vi "bigcryo-T-full.vi"() -> (2 "VTI [K]":dbl=1.4652, 3 "Spl [K]":dbl=1.6452)   [LabVIEW 2019]
uses:
  Global 2.vi
  <vilib>/Analysis/NI_AALPro.lvlib
panel:
  out "Stable?":bool
  out "read buffer":string
  in  "stop":bool
  out "Running Sequence":bool
  out "VTI Rate":dbl format="%#.3g"
  out "Rate":dbl format="%#.3g"
  in  "Rate":dbl
  in  "Reset Graph":bool
  in  "Ramp":bool
  in  "Go To":bool
  in  "Set Temp":dbl=1.6
  out "Range":dbl
  out "Spl":dbl(slide) scale=0.0..100.0
  out "VTI":dbl(slide) scale=0.0..100.0
  out "T":cluster{"X":dbl[], "Y":dbl[]}[](graph)=[{"X"=[158.55365709999998, 159.610163, 160.67648119999998, 161.7360579, 162.7961535, 163.85780699999998], "Y"=[1.4652, 1.4652, 1.4653, 1.4652, 1.4651, 1.4652]}, {"X"=[158.55365709999998, 159.610163, 160.67648119999998, 161.7360579, 162.7961535, 163.85780699999998], "Y"=[1.6459, 1.6456, 1.6455, 1.6454, 1.6452, 1.6452]}] caption="XY Graph"
  out "Set VTI [K]":dbl=1.2
  out "Set Spl [K]":dbl=1.6
  # "Heaters"
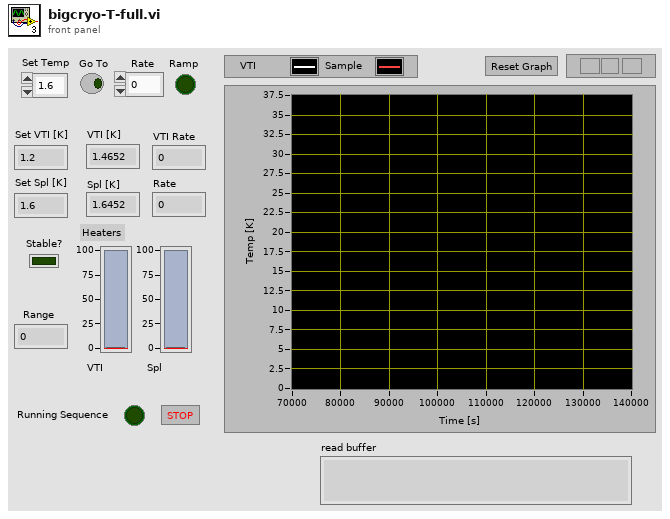
[diagram p1: front panel]
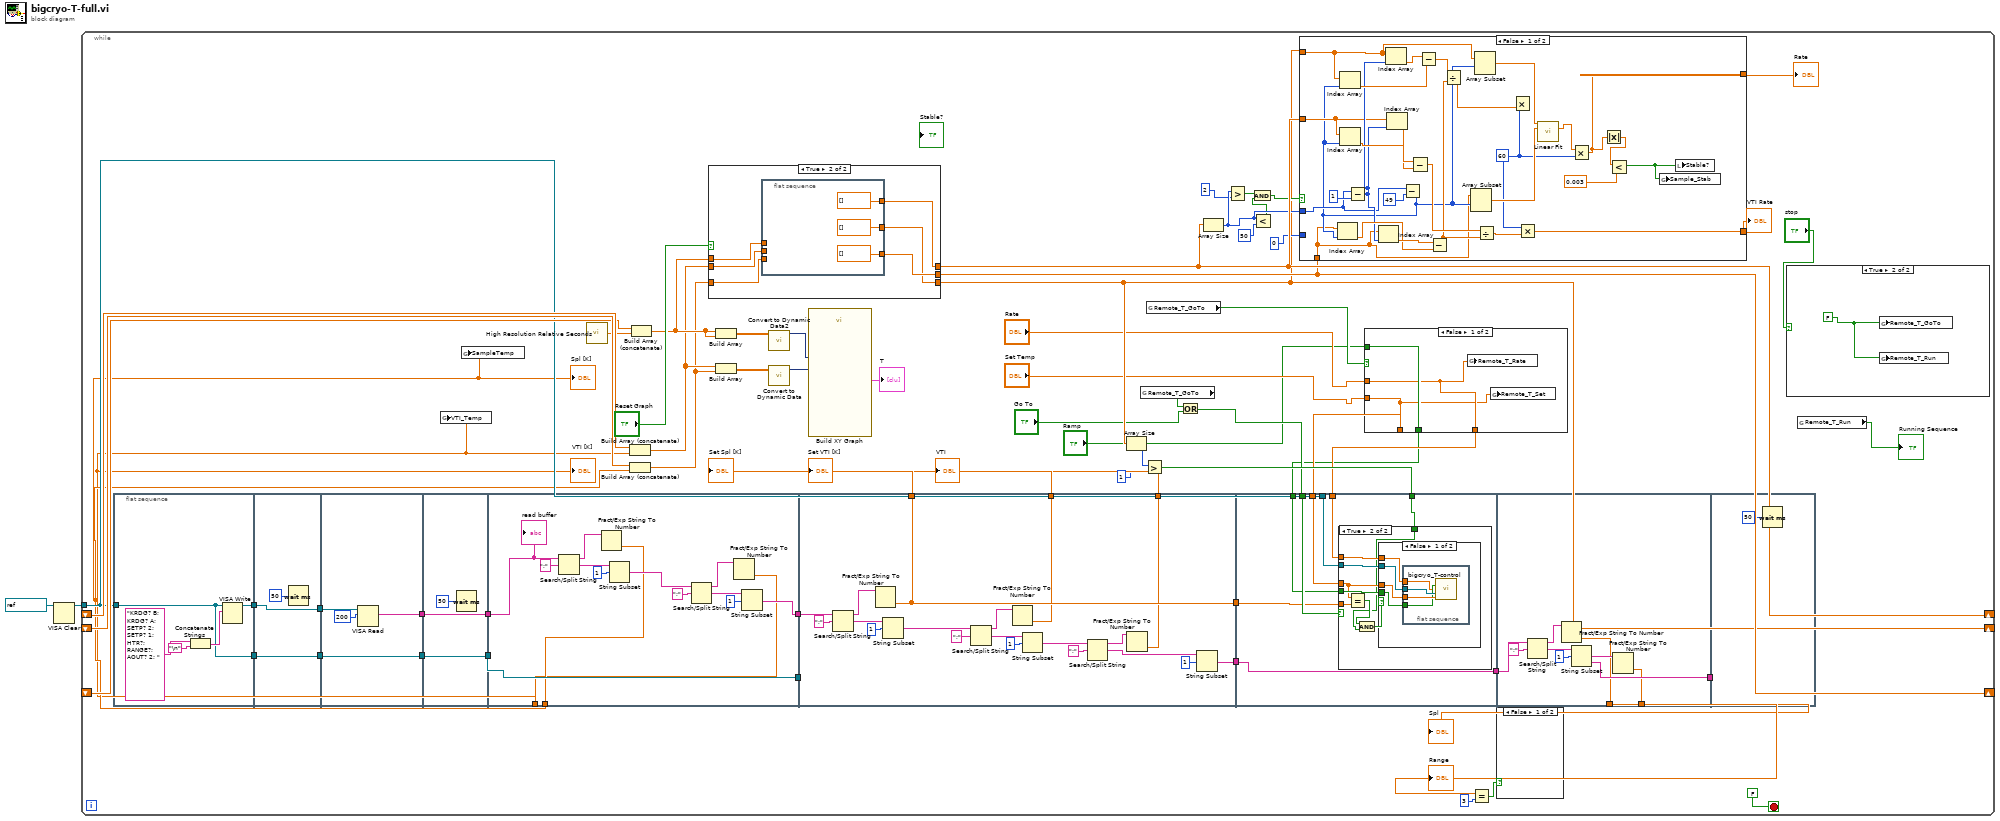
[diagram p0: block diagram]
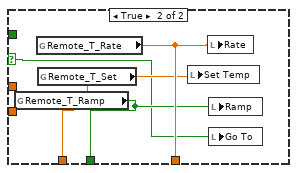
[diagram p3: hidden frame]
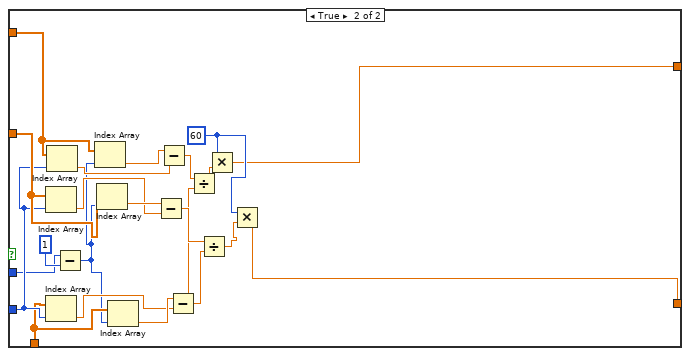
[diagram p4: hidden frame]
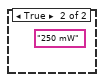
[diagram p6: hidden frame]
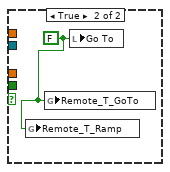
[diagram p8: hidden frame]
diagram:
  n1 = VISA Clear(VISA resource name=refnum<visa-resource-name> "COM7" ("Lakeshore Address")) -> (VISA resource name out=w2:refnum<visa-resource-name>)  [unwired: 1 in, 1 out]
  n2 = while {
    tunnel: w2 -> [w34]
    shift-right: [w19] -> _
    shift-left: _ -> [w62]
    shift-right: [w31] -> _
    shift-left: _ -> [w61]
    shift-right: [w28] -> _
    shift-left: _ -> [w59]
    stop <- FALSE stop-if-true
    n3 = flat-sequence {
      tunnel: w34 -> [w138]
      tunnel: [w138] -> w44
      tunnel: [w137] -> w41
      tunnel: w44 -> [w144]
      tunnel: [w144] -> w43
      tunnel: [w142] -> w42
      tunnel: w41 -> [w142]
      tunnel: [w148] -> w50
      tunnel: w43 -> [w148]
      tunnel: w42 -> [w146]
      tunnel: [w145] -> w38
      tunnel: [w151] -> w67
      tunnel: w50 -> [w151]
      tunnel: [w149] -> w39
      tunnel: w38 -> [w149]
      tunnel: w67 -> [w165]
      tunnel: [w152] -> w15
      tunnel: [w153] -> w16
      tunnel: [w165] -> w63
      tunnel: [w154] -> w40
      tunnel: w39 -> [w156]
      tunnel: [w184] -> w36
      tunnel: [w183] -> w33
      tunnel: [w182] -> w53
      tunnel: [w176] -> w65
      tunnel: [w183] -> w66
      tunnel: w40 -> [w167]
      tunnel: w63 -> [_]
      tunnel: w36 -> [w192]
      tunnel: [w192] -> w35
      tunnel: w12 -> [w191]
      tunnel: w34 -> [w190]
      tunnel: w7 -> [w189]
      tunnel: w5 -> [w188]
      tunnel: w9 -> [w187]
      tunnel: w33 -> [w186]
      tunnel: w17 -> [w185]
      tunnel: [w217] -> w37
      tunnel: [w216] -> w32
      tunnel: w35 -> [w210]
      tunnel: [w215] -> w45
      tunnel: w37 -> [_]
      frame #0 {
        n4 = Concatenate Strings("KRDG? B; KRDG? A; SETP? 2; SETP? 1; HTR?; RANGE?; AOUT? 2; " ("write buffer"), "\n") -> (w139:string)
        n5 = VISA Write(VISA resource name=w138, write buffer=w139) -> (VISA resource name out=w137:refnum<visa-resource-name>)  [unwired: 1 in, 2 out]
      }
      frame #1 {
        n6 = Wait (ms)(milliseconds to wait=50) -> ()  [unwired: 1 out]
      }
      frame #2 {
        n7 = VISA Read(VISA resource name=w146, byte count=u32 200) -> (read buffer=w145:string)  [unwired: 1 in, 3 out]
      }
      frame #3 {
        n8 = Wait (ms)(milliseconds to wait=50) -> ()  [unwired: 1 out]
      }
      frame #4 {
        n9 = Search/Split String(string=w156, search string/char (-)=";") -> (substring before match=w161:string, match + rest of string=w163:string)  [unwired: 1 in, 1 out]
        n10 = Fract/Exp String To Number(string=w161) -> (number=w153:dbl)  [unwired: 3 in, 1 out]
        n11 = String Subset(string=w163, offset (0)=u32 1 ("byte count")) -> (substring=w155:string)  [unwired: 1 in]
        n12 = Search/Split String(string=w155, search string/char (-)=";") -> (substring before match=w157:string, match + rest of string=w159:string)  [unwired: 1 in, 1 out]
        n13 = Fract/Exp String To Number(string=w157) -> (number=w152:dbl)  [unwired: 3 in, 1 out]
        n14 = String Subset(string=w159, offset (0)=u32 1 ("byte count")) -> (substring=w154:string)  [unwired: 1 in]
        "read buffer" <- w156
      }
      frame #5 {
        n15 = Search/Split String(string=w167, search string/char (-)=";") -> (substring before match=w166:string, match + rest of string=w169:string)  [unwired: 1 in, 1 out]
        n16 = Fract/Exp String To Number(string=w166) -> (number=w183:dbl)  [unwired: 3 in, 1 out]
        n17 = String Subset(string=w169, offset (0)=u32 1 ("byte count")) -> (substring=w172:string)  [unwired: 1 in]
        n18 = Search/Split String(string=w172, search string/char (-)=";") -> (substring before match=w171:string, match + rest of string=w174:string)  [unwired: 1 in, 1 out]
        n19 = Fract/Exp String To Number(string=w171) -> (number=w176:dbl)  [unwired: 3 in, 1 out]
        n20 = String Subset(string=w174, offset (0)=u32 1 ("byte count")) -> (substring=w178:string)  [unwired: 1 in]
        n21 = Search/Split String(string=w178, search string/char (-)=";") -> (substring before match=w177:string, match + rest of string=w180:string)  [unwired: 1 in, 1 out]
        n22 = Fract/Exp String To Number(string=w177) -> (number=w182:dbl)  [unwired: 3 in, 1 out]
        n23 = String Subset(string=w180, offset (0)=u32 1 ("byte count")) -> (substring=w184:string)  [unwired: 1 in]
      }
      frame #6 {
        n24 = case shown="True" w191 {
          tunnel: w190 -> [_ w200]
          tunnel: w189 -> [_ w196]
          tunnel: w188 -> [_ w199]
          tunnel: w187 -> [_ w198]
          tunnel: w186 -> [_ w197]
          tunnel: w185 -> [_ w194]
          frame False {
          }
          frame True {
            n25 = Equal?(x=w196, y=w197) -> (x = y?=w195:bool)
            n26 = And(x=w195, y=w194) -> (x .and. y?=w193:bool)
            n27 = case shown="False" w193 {
              tunnel: w200 -> [w204 _]
              tunnel: w196 -> [w203 _]
              tunnel: w199 -> [w202 _]
              tunnel: w198 -> [w201 _]
              frame False {
                n28 = flat-sequence {
                  tunnel: w204 -> [w208]
                  tunnel: w203 -> [w207]
                  tunnel: w202 -> [w206]
                  tunnel: w201 -> [w205]
                  frame #0 {
                    n29 = call "bigcryo_T-control.vi"("Ramp Mode"=w206, "Rate  [K/min]"=w205, "VISA resource name out"=w208, "Set Sample Temp [K]"=w207) -> ()  [unwired: 12 in]
                  }
                }
              }
              frame True {
                w209 = FALSE
                n30 = global write "Global 2.vi" "Remote_T_Ramp"(w209) -> ()
                n31 = global write "Global 2.vi" "Remote_T_GoTo"(w209) -> ()
                n32 = local write "Go To"(w209) -> ()
              }
            }
          }
        }
      }
      frame #7 {
        n33 = Search/Split String(string=w210, search string/char (-)=";") -> (substring before match=w211:string, match + rest of string=w213:string)  [unwired: 1 in, 1 out]
        n34 = Fract/Exp String To Number(string=w211) -> (number=w215:dbl)  [unwired: 3 in, 1 out]
        n35 = String Subset(string=w213, offset (0)=u32 1 ("byte count")) -> (substring=w217:string)  [unwired: 1 in]
        n36 = Fract/Exp String To Number(string=w217) -> (number=w216:dbl)  [unwired: 3 in, 1 out]
      }
      frame #8 {
        n37 = Wait (ms)(milliseconds to wait=50) -> ()  [unwired: 1 out]
      }
    }
    n38 = global write "Global 2.vi" "VTI_Temp"(w15) -> ()
    n39 = global write "Global 2.vi" "SampleTemp"(w16) -> ()
    n40 = call <vilib>:"High Resolution Relative Seconds.vi"() -> ("relative seconds"=w58:dbl)
    n41 = Build Array (concatenate)(w61, w15) -> (w47:dbl[])
    n42 = Build Array (concatenate)(w62, w16) -> (w46:dbl[])
    n43 = Build Array (concatenate)(w59, w58) -> (w48:dbl[])
    n44 = case shown="True" "Reset Graph" {
      tunnel: w48 -> [w127 w133]
      tunnel: [w127 w132] -> w28
      tunnel: w47 -> [w126 w131]
      tunnel: [w126 w130] -> w31
      tunnel: w46 -> [w125 w129]
      tunnel: [w125 w128] -> w19
      frame False {
      }
      frame True {
        n45 = flat-sequence {
          tunnel: w133 -> [_]
          tunnel: w131 -> [_]
          tunnel: w129 -> [_]
          tunnel: [dbl[] []] -> w130
          tunnel: [dbl[] []] -> w132
          tunnel: [dbl[] []] -> w128
          frame #0 {
          }
        }
      }
    }
    n46 = Build Array(w48, w48) -> (w55:dbl[][])
    n47 = Build Array(w47, w46) -> (w57:dbl[][])
    n48 = call "Convert to Dynamic Data2"("2D Array"=w55) -> ("Dynamic Data Type"=w54:dynamicdata)  [unwired: 3 in]
    n49 = call "Convert to Dynamic Data"("2D Array"=w57) -> ("Dynamic Data Type"=w56:dynamicdata)  [unwired: 3 in]
    n50 = call "Build XY Graph"("Y Input"=w56, "X Input"=w54) -> ("XY Graph"=→"T":cluster{"X":dbl[], "Y":dbl[]}[])  [unwired: 8 in, 1 out]
    n51 = Array Size(array=w19) -> (size(s)=w20:i32)
    n52 = global read "Global 2.vi" "Remote_T_GoTo"() -> (w14:bool)
    n53 = Greater?(x=w20, y=1) -> (0:w17:bool)
    n54 = global read "Global 2.vi" "Remote_T_GoTo"() -> (w11:bool)
    n55 = Or(x=w14, y="Go To") -> (x .or. y?=w12:bool)
    n56 = Array Size(array=w31) -> (size(s)=w25:i32)
    n57 = Greater?(x=w25, y=2) -> (0:w27:bool)
    n58 = Less?(x=w25, y=50) -> (x < y?=w23:bool)
    n59 = And(x=w27, y=w23) -> (x .and. y?=w26:bool)
    n60 = case shown="False" w26 {
      tunnel: w31 -> [w87 w124]
      tunnel: 0 -> [_ w123]
      tunnel: w25 -> [w89 w107]
      tunnel: w28 -> [w84 w121]
      tunnel: w19 -> [w86 w122]
      tunnel: [w78 w105] -> w22
      tunnel: [w90 w104] -> w21
      frame False {
        w81 = 60
        n61 = Subtract(x=w89, y=1) -> (x-y=w91:i32)
        n62 = Index Array(array=w84, index=w91) -> (element=w103:dbl)
        n63 = Index Array(array=w86, index=w91) -> (element=w99:dbl)
        n64 = Index Array(array=w87, index=w91) -> (element=w101:dbl)
        n65 = Subtract(x=w89, y=49) -> (x-y=w85:i32)
        n66 = Index Array(array=w84, index=w85) -> (element=w102:dbl)
        n67 = Index Array(array=w86, index=w85) -> (element=w98:dbl)
        n68 = Index Array(array=w87, index=w85) -> (element=w100:dbl)
        n69 = Subtract(x=w101, y=w100) -> (x-y=w96:dbl)
        n70 = Subtract(x=w99, y=w98) -> (x-y=w97:dbl)
        n71 = Subtract(x=w103, y=w102) -> (x-y=w95:dbl)
        n72 = Divide(x=w97, y=w95) -> (x/y=w94:dbl)
        n73 = Array Subset(array=w84, index=w85) -> (w82:dbl[])  [unwired: 1 in]
        n74 = Array Subset(array=w86, index=w85) -> (w83:dbl[])  [unwired: 1 in]
        n75 = Divide(x=w96, y=w95) -> (x/y=w93:dbl)
        n76 = Multiply(x=w81, y=w94) -> ()  [unwired: 1 out]
        n77 = Multiply(x=w81, y=w93) -> (x*y=w90:dbl)
        n78 = call <vilib>:"Linear Fit.vi"("Y"=w83, "X"=w82) -> ("slope"=w80:dbl)  [unwired: 9 in, 4 out]
        n79 = Multiply(x=w80, y=w81) -> (x*y=w78:dbl)
        n80 = Absolute Value(x=w78) -> (abs(x)=w77:dbl)
        n81 = Less?(x=w77, y=0.003) -> (x < y?=w76:bool)
        n82 = global write "Global 2.vi" "Sample_Stab"(w76) -> ()
        n83 = local write "Stable?"(w76) -> ()
      }
      frame True {
        w110 = 60
        n84 = Index Array(array=w124, index=w123) -> (element=w117:dbl)
        n85 = Index Array(array=w121, index=w123) -> (element=w119:dbl)
        n86 = Index Array(array=w122, index=w123) -> (element=w115:dbl)
        n87 = Subtract(x=w107, y=1) -> (x-y=w106:i32)
        n88 = Index Array(array=w122, index=w106) -> (element=w116:dbl)
        n89 = Index Array(array=w124, index=w106) -> (element=w118:dbl)
        n90 = Index Array(array=w121, index=w106) -> (element=w120:dbl)
        n91 = Subtract(x=w118, y=w117) -> (x-y=w113:dbl)
        n92 = Subtract(x=w116, y=w115) -> (x-y=w114:dbl)
        n93 = Subtract(x=w120, y=w119) -> (x-y=w112:dbl)
        n94 = Divide(x=w114, y=w112) -> (x/y=w111:dbl)
        n95 = Divide(x=w113, y=w112) -> (x/y=w109:dbl)
        n96 = Multiply(x=w110, y=w111) -> (x*y=w105:dbl)
        n97 = Multiply(x=w110, y=w109) -> (x*y=w104:dbl)
      }
    }
    "Rate" <- w22
    "VTI Rate" <- w21
    n98 = case shown="False" w11 {
      selector: w11 -> [_ w72]
      tunnel: "Rate" -> [w70 _]
      tunnel: [w70 w75] -> w9
      tunnel: "Set Temp" -> [w69 _]
      tunnel: [w69 w74] -> w7
      tunnel: "Ramp" -> [w71 _]
      tunnel: [w71 w73] -> w5
      frame False {
        n99 = global write "Global 2.vi" "Remote_T_Rate"(w70) -> ()
        n100 = global write "Global 2.vi" "Remote_T_Set"(w69) -> ()
      }
      frame True {
        n101 = global read "Global 2.vi" "Remote_T_Ramp"() -> (w73:bool)
        n102 = global read "Global 2.vi" "Remote_T_Rate"() -> (w75:dbl)
        n103 = global read "Global 2.vi" "Remote_T_Set"() -> (w74:dbl)
        n104 = local write "Set Temp"(w74) -> ()
        n105 = local write "Rate"(w75) -> ()
        n106 = local write "Ramp"(w73) -> ()
        n107 = local write "Go To"(w72) -> ()
      }
    }
    n108 = Equal?(x=w45, y=3) -> (x = y?=w51:bool)
    n109 = case shown="False" w51 {
      frame False {
      }
      frame True {
        (unwired) "250 mW"
      }
    }
    n110 = case shown="True" "stop" {
      frame False {
      }
      frame True {
        w68 = FALSE
        n111 = global write "Global 2.vi" "Remote_T_GoTo"(w68) -> ()
        n112 = global write "Global 2.vi" "Remote_T_Run"(w68) -> ()
      }
    }
    n113 = global read "Global 2.vi" "Remote_T_Run"() -> (→"Running Sequence":bool)
    "Spl [K]" <- w16
    "VTI [K]" <- w15
    "Set Spl [K]" <- w66
    "Set VTI [K]" <- w65
    "VTI" <- w53
    "Spl" <- w32
    "Range" <- w45
  }
